vi "ROI_Processing.vi"(6 "Pixel Size(um)":dbl, 7 "Histogram Mode":enum16{"ROI", "Image"}(ring), 8 "error in (no error)":errorcluster, 9 "ROI":T1, 10 "Image Dst Out":T2, 11 "WaveformGraph in":refnum<vi>) -> (0 "error out":errorcluster, 3 "ROI Pixel Statistics":T3 {"Min" format="%.2f"; "Std Dev" format="%.2f"; "Mean" format="%.2f"; "Max" format="%.2f"})   [LabVIEW 2023, in "CameraLibrary.lvlib" / "Camera_Controller.lvlib"]
uses:
  Camera_Controller.lvlib
  <vilib>/vision/Image Controls.llb/IMAQ Image.ctl
  <vilib>/vision/NI_Vision_Development_Module.lvlib
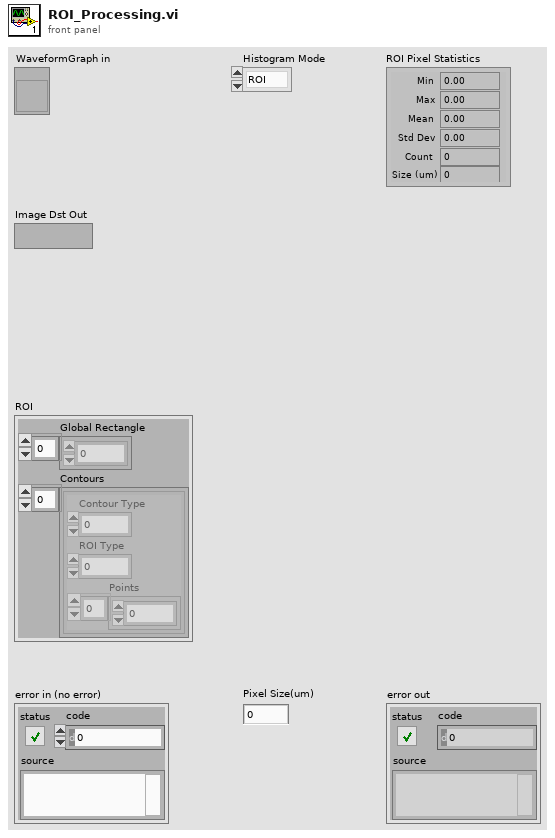
[diagram p1: front panel]
types:
  T1 = cluster{"Global Rectangle":i32[], "Contours":cluster{"Contour Type":u32, "ROI Type":u32, "Points":i32[]}[]}
  T2 = typedef "IMAQ Image.ctl" = refnum<image>
  T3 = cluster{"Min":sgl, "Max":sgl, "Mean":sgl, "Std Dev":sgl, "Count":i32, "Size (um)":i32}
  T4 = cluster{"Min":sgl, "Max":sgl, "Mean":sgl, "Std Dev":sgl, "Count":i32}
  T5 = cluster{"Starting Value":sgl, "Incremental Value":sgl, "Histogram":u32[]}
  T6 = cluster{"Min":sgl, "Max":sgl, "Mean":sgl, "Std Dev":sgl, "Count":i32, dbl}
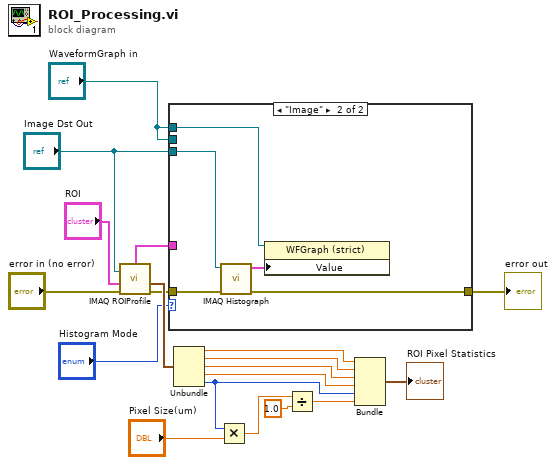
[diagram p0: block diagram]
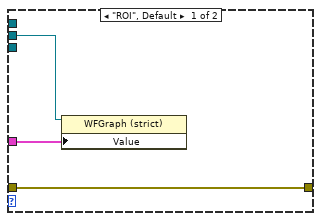
[diagram p2: hidden frame]
diagram:
  n1 = call "IMAQ ROIProfile"("error in (no error)"="error in (no error)", "ROI Descriptor"="ROI", "Image"="Image Dst Out") -> ("ROI Pixel Statistics"=w5:T4, "error out"=w4:errorcluster, "ROI Graph"=w3:cluster{"x0":sgl, "dx":sgl, "Pixels Line":sgl[]})  [unwired: 1 in, 2 out]
  n2 = case shown="\"Image\"" "Histogram Mode" {
    tunnel: [w21 w26] -> w15
    tunnel: w4 -> [w21 w27]
    tunnel: w3 -> [w22 _]
    tunnel: "Image Dst Out" -> [_ w24]
    tunnel: "WaveformGraph in" -> [w20 _]
    tunnel: "WaveformGraph in" -> [_ w23]
    frame "ROI", Default {
      n3 = property class="WFGraph (strict)"(reference=w20, "Value"=w22) -> ()  [unwired: 1 in, 2 out]
    }
    frame "Image" {
      n4 = call "IMAQ Histograph"("error in (no error)"=w27, "Image"=w24) -> ("error out"=w26:errorcluster, "Histogram Graph"=w25:T5)  [unwired: 6 in, 2 out]
      n5 = property class="WFGraph (strict)"(reference=w23, "Value"=w25) -> ()  [unwired: 1 in, 2 out]
    }
  }
  "error out" <- w15
  n6 = Unbundle(w5) -> ("Min"=w9:sgl, "Max"=w8:sgl, "Mean"=w7:sgl, "Std Dev"=w6:sgl, "Count"=w10:i32)
  n7 = Multiply(x=w10, y="Pixel Size(um)") -> (x*y=w12:dbl)
  n8 = Divide(x=w12, y=1.0) -> (x/y=w13:dbl)
  n9 = Bundle("Min"=w9, "Max"=w8, "Mean"=w7, "Std Dev"=w6, "Count"=w10, w13) -> (→"ROI Pixel Statistics":T6)  [unwired: 1 in]
